vi "Utilities_Startup_Folder_Setup.vi"   [LabVIEW 2020]
uses:
  <vilib>/MakerHub/Toolbox/LMH-Toolbox.lvlib
types:
  T1 = enum16{"open", "open or create", "create or replace", "create", "open (read-only)"}
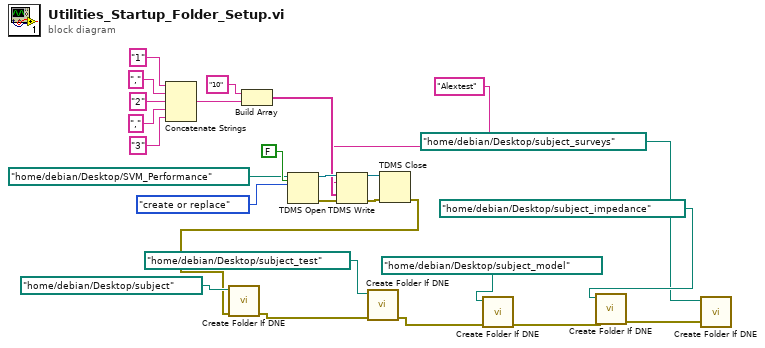
[diagram p0: block diagram]
diagram:
  n1 = Concatenate Strings("1" ("string"), "," ("string"), "2" ("string"), "," ("string"), "3" ("string")) -> (w14:string)
  n2 = Build Array("10", w14) -> (w13:string[])
  n3 = TDMS Open(5:FALSE ("create index file? (T)"), 10:T1."create or replace" ("operation (0:open)"), 11:path "/home/debian/Desktop/SVM_Performance" ("base path")) -> (0:w23:errorcluster, 3:w22:refnum<k34>)  [unwired: 4 in]
  n4 = TDMS Write(0:w22, 5:"Alextest" ("group name in (Untitled)"), 9:w13, 11:w23) -> (4:w25:refnum<k34>, 15:w26:errorcluster)  [unwired: 2 in, 2 out]
  n5 = TDMS Close(8:w26, 11:w25) -> (0:w9:errorcluster)  [unwired: 1 out]
  n6 = call <vilib>:"Create Folder If DNE.vi"("Error In"=w9, "Folder Path"=path "/home/debian/Desktop/subject" ("base path")) -> ("Error Out"=w8:errorcluster)  [unwired: 8 in, 1 out]
  n7 = call <vilib>:"Create Folder If DNE.vi"("Error In"=w8, "Folder Path"=path "/home/debian/Desktop/subject_test" ("base path")) -> ("Error Out"=w7:errorcluster)  [unwired: 8 in, 1 out]
  n8 = call <vilib>:"Create Folder If DNE.vi"("Error In"=w7, "Folder Path"=path "/home/debian/Desktop/subject_model" ("base path")) -> ("Error Out"=w4:errorcluster)  [unwired: 8 in, 1 out]
  n9 = call <vilib>:"Create Folder If DNE.vi"("Error In"=w4, "Folder Path"=path "/home/debian/Desktop/subject_impedance" ("base path")) -> ("Error Out"=w2:errorcluster)  [unwired: 8 in, 1 out]
  n10 = call <vilib>:"Create Folder If DNE.vi"("Error In"=w2, "Folder Path"=path "/home/debian/Desktop/subject_surveys") -> ()  [unwired: 8 in, 2 out]
